vi "Save Load.vi"(6 "error in":errorcluster, 7 "Sub-panel VI names":string[](array[string]), 8 "Temp file path":path=path "D:/control db/control software/Control vi/Temp control/save all temp.txt", 9 "Beamline Section":T1, 10 "Save Load Method":T2, 11 "Sub-panel VI paths array":path[](array[path])) -> (0 "Save Load Error Array Out":errorcluster[](array[cluster]), 2 "Settings Data":cluster{"Name":string, "Variant Data":variant}[](array[cluster]), 3 "Settings Text":string, 4 "enum conversion error array":errorcluster[](array[cluster]))   [LabVIEW 2016, in "Save Load.lvlib"]
doc: "Takes a vi and saves or loads set values depending on which cluster value is chosen"
uses:
  Save Load.lvlib
  save load method.ctl
  beamline selection.ctl
  save or load.ctl
  file or temp.ctl
  all or current.ctl
  main.lvlib
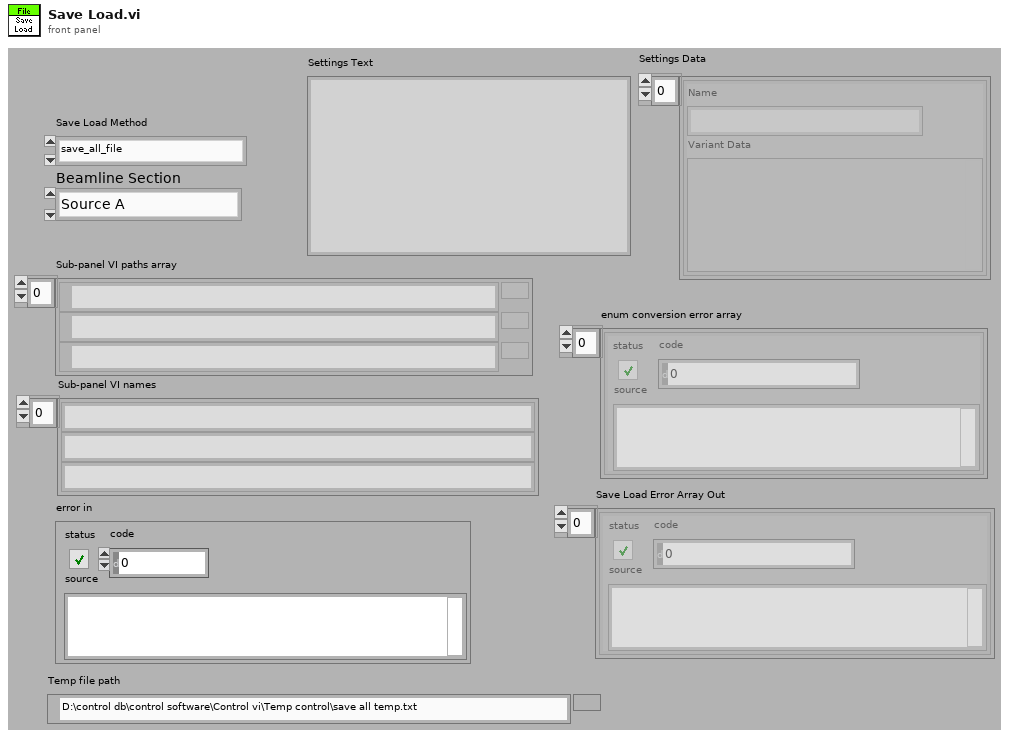
[diagram p1: front panel]
types:
  T1 = typedef "main.lvlib/beamline selection.ctl" = enum16{"Source A", "Source B", "Low Energy End", "High Energy End", "Transmission", "R30", "R45"}
  T2 = typedef "Save Load.lvlib/save load method.ctl" = enum16{"save_all_file", "save_all_temp", "save_curr_file", "save_curr_temp", "load_all_file", "load_all_temp", "load_curr_file", "load_curr_temp"}
  T3 = typedef "Save Load.lvlib/all or current.ctl" = enum16{"current", "all"}
  T4 = typedef "Save Load.lvlib/file or temp.ctl" = enum16{"file", "temp"}
  T5 = typedef "Save Load.lvlib/save or load.ctl" = enum16{"save", "load"}
  T6 = cluster{"format string":string, "format string":string}
  T7 = cluster{"format string":string, "format string":string}[]
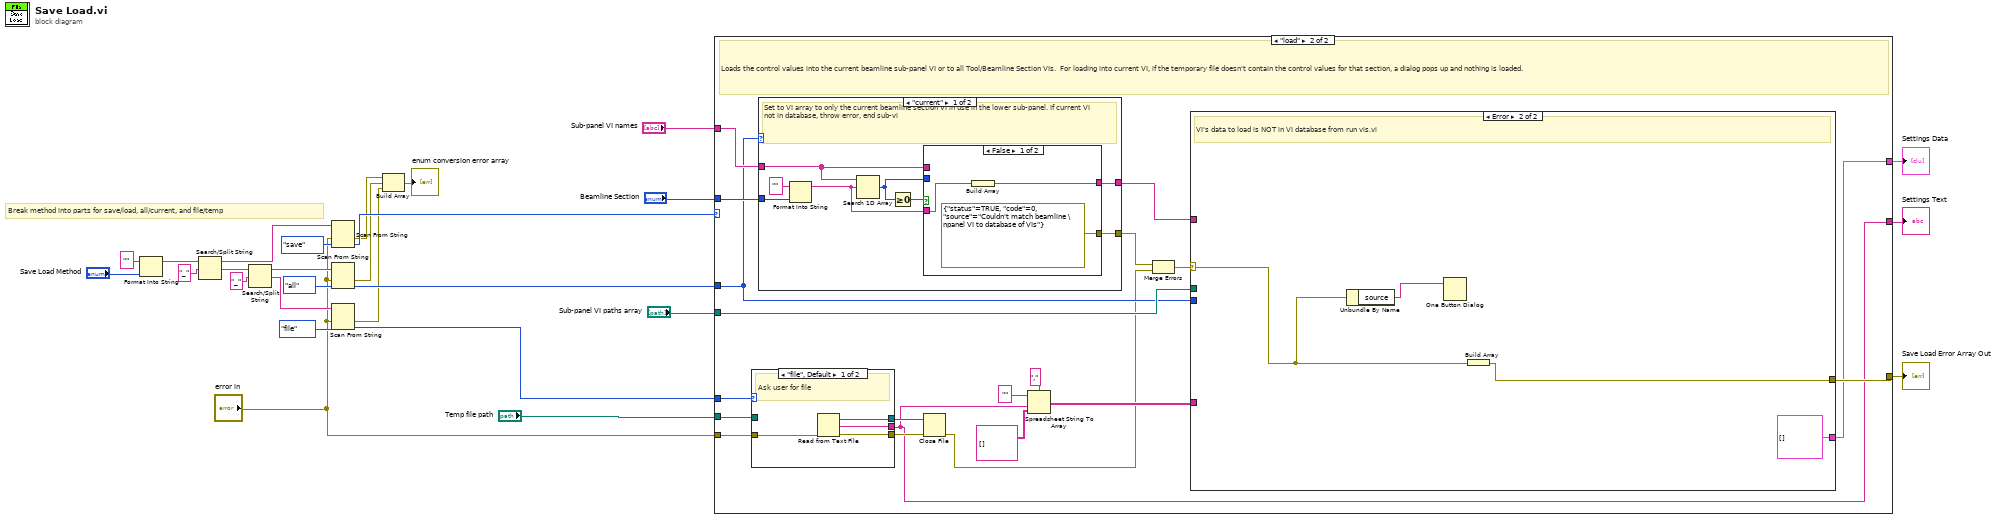
[diagram p0: block diagram]
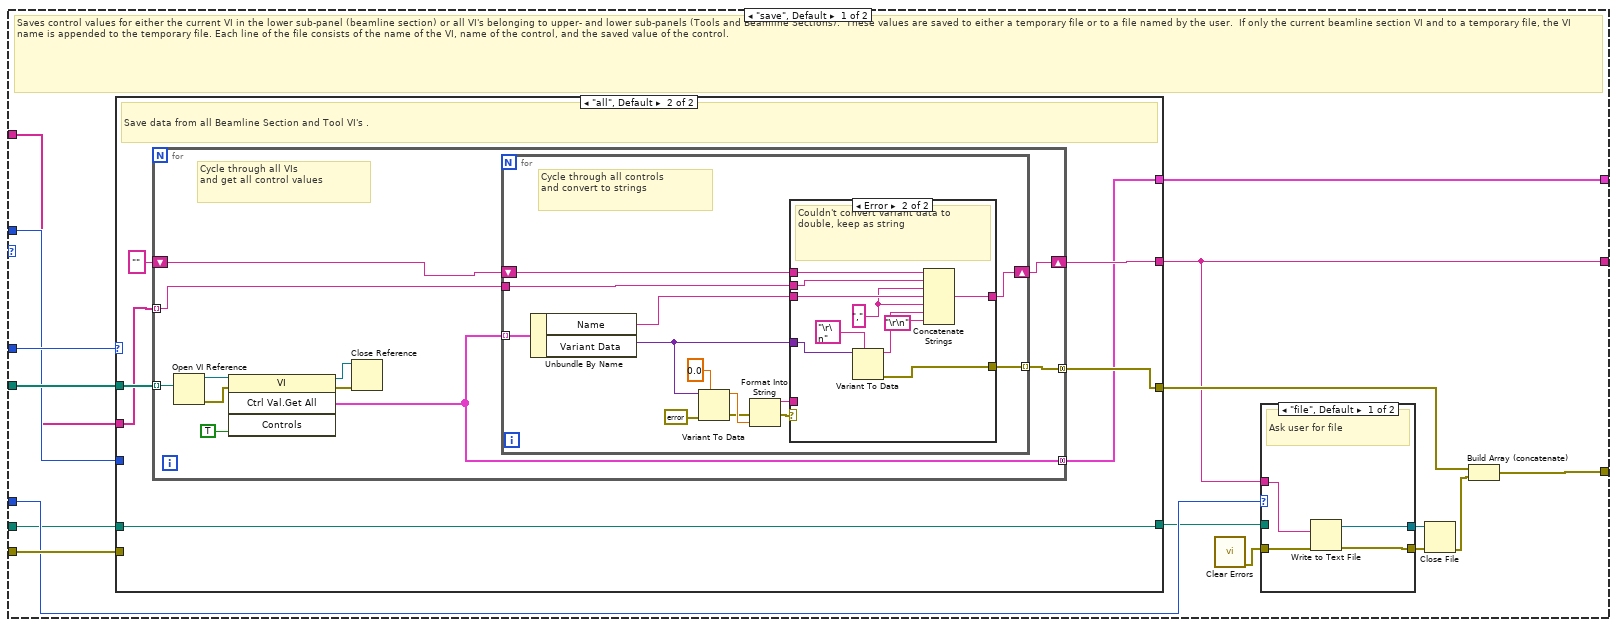
[diagram p2: hidden frame]
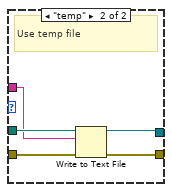
[diagram p3: hidden frame]
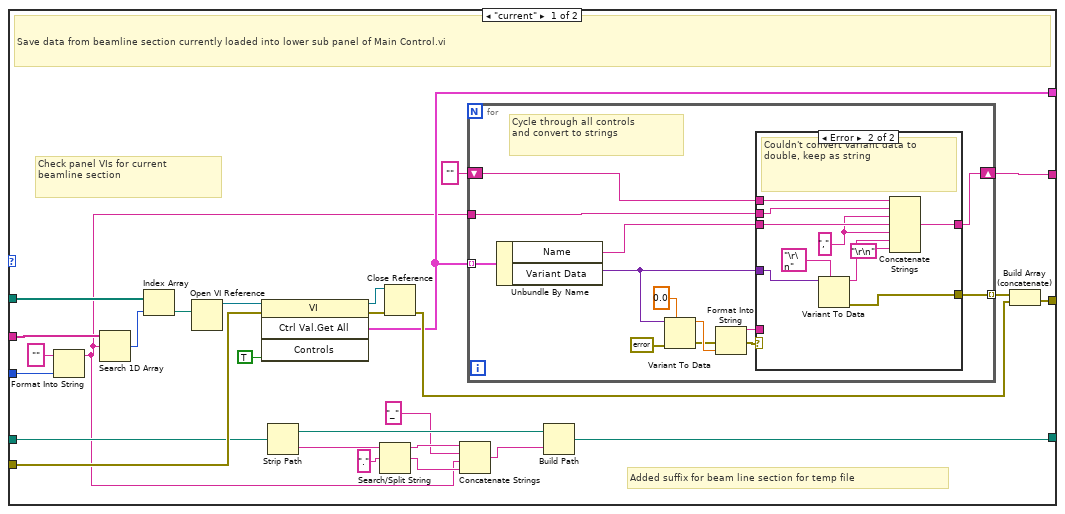
[diagram p4: hidden frame]
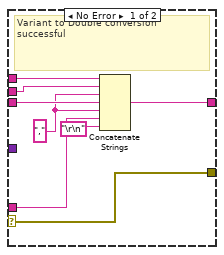
[diagram p5: hidden frame]
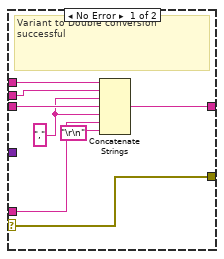
[diagram p6: hidden frame]
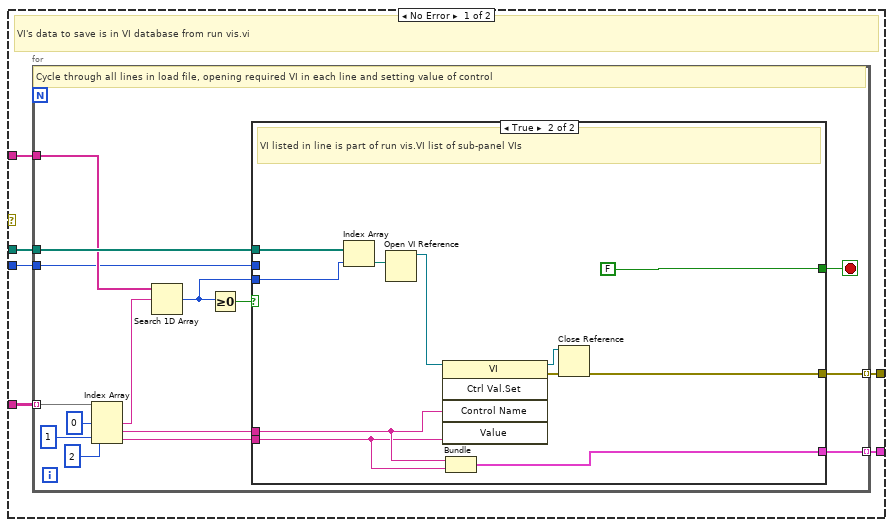
[diagram p7: hidden frame]
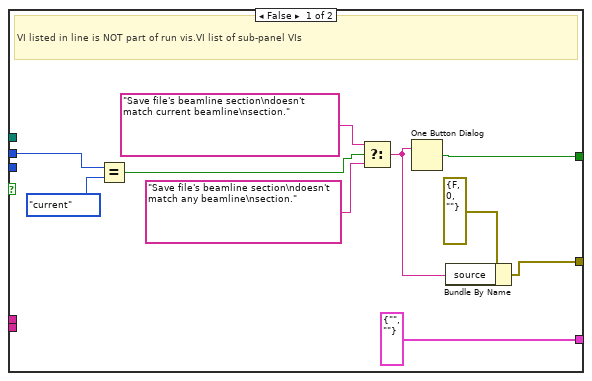
[diagram p8: hidden frame]
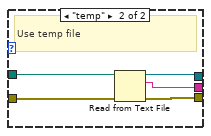
[diagram p9: hidden frame]
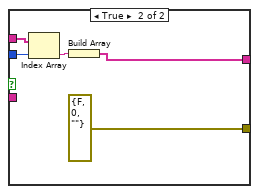
[diagram p10: hidden frame]
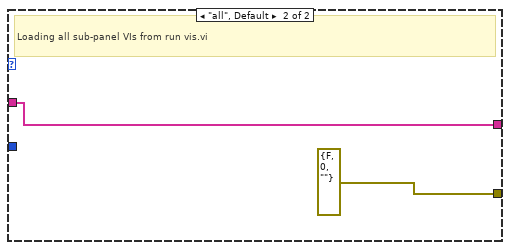
[diagram p11: hidden frame]
diagram:
  # "Break method into parts for save/load, all/current, and file/temp"
  n1 = Format Into String(initial string="", "Save Load Method") -> (resulting string=w24:string)  [unwired: 2 in, 1 out]
  n2 = Search/Split String(string=w24, search string/char (-)="_") -> (substring before match=w19:string, match + rest of string=w25:string)  [unwired: 1 in, 1 out]
  n3 = Search/Split String(string=w25, search string/char (-)="_") -> (substring before match=w18:string, match + rest of string=w17:string)  [unwired: 1 in, 1 out]
  n4 = Scan From String(input string=w19, error in="error in", default 1=save_or_load."save") -> (error out=w13:errorcluster, output 1=w15:T5)  [unwired: 2 in, 2 out]
  n5 = Scan From String(input string=w18, error in="error in", default 1=all_or_current."all") -> (error out=w12:errorcluster, output 1=w14:T3)  [unwired: 2 in, 2 out]
  n6 = Scan From String(input string=w17, error in="error in", default 1=file_or_temp."file") -> (error out=w11:errorcluster, output 1=w9:T4)  [unwired: 2 in, 2 out]
  n7 = Build Array(w13, w12, w11) -> (→"enum conversion error array":errorcluster[])
  n8 = case shown="\"load\"" w15 {
    tunnel: w14 -> [w43 w163]
    tunnel: w9 -> [w30 w179]
    tunnel: "error in" -> [w37 w178]
    tunnel: "Temp file path" -> [w29 w177]
    tunnel: "Sub-panel VI names" -> [w38 w173]
    tunnel: "Sub-panel VI paths array" -> [w40 w168]
    tunnel: "Beamline Section" -> [w39 w174]
    tunnel: [w33 w167] -> w3
    tunnel: [w32 w166] -> w2
    tunnel: [w31 w164] -> w1
    frame "save", Default {
      # "Saves control values for either the current VI in the lower sub-panel (beamline section) or all VI's belonging to upper- and lower sub-panels (Tools and Beamline Sections).  These values are saved to either a temporary file or to a file named by the user.  If only the current beamline section VI and to a temporary file, the VI name is appended to the temporary file. Each line of the file consists of the name of the VI, name of the control, and the saved value of the control."
      n9 = case shown="\"all\", Default" w43 {
        tunnel: w40 -> [w75 w117]
        tunnel: w39 -> [w79 _]
        tunnel: w38 -> [w77 w115]
        tunnel: w37 -> [w63 _]
        tunnel: [w65 w113] -> w34
        tunnel: [w68 w114] -> w32
        tunnel: [w64 w112] -> w31
        tunnel: w29 -> [w62 w111]
        tunnel: [w53 w111] -> w28
        frame "current" {
          # "Check panel VIs for current \nbeamline section"
          # "Added suffix for beam line section for temp file"
          # "Save data from beamline section currently loaded into lower sub panel of Main Control.vi"
          n10 = Format Into String(initial string="", w79) -> (resulting string=w54:string)  [unwired: 2 in, 1 out]
          n11 = Search 1D Array(1D array=w77, element=w54) -> (index of element=w76:i32)  [unwired: 1 in]
          n12 = Index Array(array=w75, index=w76) -> (element=w74:path)
          n13 = Open VI Reference(vi path=w74) -> (vi reference=w73:refnum<vi>)  [unwired: 5 in, 1 out]
          n14 = invoke class="VI" method="Ctrl Val.Get All"(reference=w73, error in=w63, "Controls"=TRUE) -> (reference out=w70:refnum<vi>, error out=w71:errorcluster, "Get All Control Values Variant"=w64:cluster{"Name":string, "Variant Data":variant}[])  [unwired: 1 in, 1 out]
          n15 = Strip Path(path=w62) -> (stripped path=w57:path, name=w61:string)
          n16 = Search/Split String(string=w61, search string/char (-)=".") -> (substring before match=w59:string, match + rest of string=w56:string)  [unwired: 1 in, 1 out]
          n17 = Close Reference(reference=w70, error in (no error)=w71) -> (error out=w66:errorcluster)
          n18 = Concatenate Strings(w59, "_" ("string"), w54, w56) -> (w58:string)
          n19 = for {
            tunnel: w64 -> [w92] mode=indexing
            shift-right: [w86] -> w68
            shift-left: "" -> [w91]
            tunnel: [w82] -> w67 mode=indexing
            tunnel: w54 -> [w81]
            # "Cycle through all controls\nand convert to strings"
            # "Cycle through all the controls on the current beamline section panel"
            n20 = Unbundle By Name(w92) -> ("Name"=w90:string, "Variant Data"=w80:variant)
            n21 = Variant To Data(error in=errorcluster {"status"=FALSE, "code"=0, "source"=""} ("error out"), type=0.0, Variant=w80) -> (data=w88:dbl, error out=w85:errorcluster)
            n22 = Format Into String(error in=w85, w88) -> (resulting string=w87:string, error out=w83:errorcluster)  [unwired: 2 in]
            n23 = case shown="Error" w83 {
              selector: w83 -> [w96 _]
              tunnel: [w99 w105] -> w86
              tunnel: w91 -> [w95 w103]
              tunnel: w90 -> [w98 w106]
              tunnel: w87 -> [w97 _]
              tunnel: w80 -> [_ w109]
              tunnel: [w96 w104] -> w82
              tunnel: w81 -> [w93 w102]
              frame No Error {
                w94 = ","
                # "Variant to Double conversion successful"
                n24 = Concatenate Strings(w95, w93, w94, w98, w94, w97, "\r\n") -> (w99:string)
              }
              frame Error {
                w101 = ","
                # "Couldn't convert variant data to double, keep as string"
                n25 = Variant To Data(type="\r\n", Variant=w109) -> (data=w107:string, error out=w104:errorcluster)  [unwired: 1 in]
                n26 = Concatenate Strings(w103, w102, w101, w106, w101, w107, "\r\n") -> (w105:string)
              }
            }
          }
          n27 = Build Path(base path=w57, name or relative path=w58) -> (appended path=w53:path)
          n28 = Build Array (concatenate)(w67, w66) -> (w65:errorcluster[])
        }
        frame "all", Default {
          # "Save data from all Beamline Section and Tool VI's ."
          n29 = for {
            tunnel: w117 -> [w128] mode=indexing
            shift-right: [w120] -> w114
            shift-left: "" -> [w122]
            tunnel: w115 -> [w121] mode=indexing
            tunnel: [w119] -> w113 mode=concatenating
            tunnel: [w118] -> w112 mode=concatenating
            # "Cycle through all VIs\nand get all control values"
            n30 = Open VI Reference(vi path=w128) -> (vi reference=w124:refnum<vi>, error out=w123:errorcluster)  [unwired: 5 in]
            n31 = invoke class="VI" method="Ctrl Val.Get All"(reference=w124, error in=w123, "Controls"=TRUE) -> (reference out=w125:refnum<vi>, error out=w126:errorcluster, "Get All Control Values Variant"=w118:cluster{"Name":string, "Variant Data":variant}[])  [unwired: 1 in, 1 out]
            n32 = Close Reference(reference=w125, error in (no error)=w126) -> ()  [unwired: 1 out]
            n33 = for {
              tunnel: w118 -> [w141] mode=indexing
              shift-right: [w135] -> w120
              shift-left: w122 -> [w140]
              tunnel: [w131] -> w119 mode=indexing
              tunnel: w121 -> [w130]
              # "Cycle through all controls\nand convert to strings"
              n34 = Unbundle By Name(w141) -> ("Name"=w139:string, "Variant Data"=w129:variant)
              n35 = Variant To Data(error in=errorcluster {"status"=FALSE, "code"=0, "source"=""} ("error out"), type=0.0, Variant=w129) -> (data=w137:dbl, error out=w134:errorcluster)
              n36 = Format Into String(error in=w134, w137) -> (resulting string=w136:string, error out=w132:errorcluster)  [unwired: 2 in]
              n37 = case shown="Error" w132 {
                selector: w132 -> [w145 _]
                tunnel: [w148 w154] -> w135
                tunnel: w140 -> [w144 w152]
                tunnel: w139 -> [w147 w155]
                tunnel: w136 -> [w146 _]
                tunnel: w129 -> [_ w158]
                tunnel: [w145 w153] -> w131
                tunnel: w130 -> [w142 w151]
                frame No Error {
                  w143 = ","
                  # "Variant to Double conversion successful"
                  n38 = Concatenate Strings(w144, w142, w143, w147, w143, w146, "\r\n") -> (w148:string)
                }
                frame Error {
                  w150 = ","
                  # "Couldn't convert variant data to double, keep as string"
                  n39 = Variant To Data(type="\r\n", Variant=w158) -> (data=w156:string, error out=w153:errorcluster)  [unwired: 1 in]
                  n40 = Concatenate Strings(w152, w151, w150, w155, w150, w156, "\r\n") -> (w154:string)
                }
              }
            }
          }
        }
      }
      n41 = call <vilib>:"Clear Errors.vi"() -> ("error out"=w36:errorcluster)  [unwired: 2 in, 5 out]
      n42 = case shown="\"file\", Default" w30 {
        tunnel: [w47 w52] -> w41
        tunnel: w36 -> [w45 w51]
        tunnel: [w46 w50] -> w42
        tunnel: w28 -> [_ w49]
        tunnel: w32 -> [w44 w48]
        frame "file", Default {
          # "Ask user for file"
          n43 = Write to Text File(text=w44, error in=w45) -> (refnum out=w47:refnum<file>, error out=w46:errorcluster)  [unwired: 2 in, 1 out]
        }
        frame "temp" {
          # "Use temp file"
          n44 = Write to Text File(file (use dialog)=w49, text=w48, error in=w51) -> (refnum out=w52:refnum<file>, error out=w50:errorcluster)  [unwired: 1 in, 1 out]
        }
      }
      n45 = Close File(refnum=w41, error in=w42) -> (error out=w35:errorcluster)  [unwired: 1 out]
      n46 = Build Array (concatenate)(w34, w35) -> (w33:errorcluster[])
    }
    frame "load" {
      # "Loads the control values into the current beamline sub-panel VI or to all Tool/Beamline Section VIs.  For loading into current VI, if the temporary file doesn't contain the control values for that section, a dialog pops up and nothing is loaded."
      n47 = case shown="\"file\", Default" w179 {
        tunnel: [w229 w234] -> w175
        tunnel: [w228 w233] -> w166
        tunnel: w178 -> [w226 w232]
        tunnel: [w227 w231] -> w176
        tunnel: w177 -> [_ w230]
        frame "file", Default {
          # "Ask user for file"
          n48 = Read from Text File(error in=w226) -> (refnum out=w229:refnum<file>, text=w228:string, error out=w227:errorcluster)  [unwired: 4 out]
        }
        frame "temp" {
          # "Use temp file"
          n49 = Read from Text File(file (use dialog)=w230, error in=w232) -> (refnum out=w234:refnum<file>, text=w233:string, error out=w231:errorcluster)  [unwired: 3 out]
        }
      }
      n50 = case shown="\"current\"" w163 {
        tunnel: w174 -> [w242 _]
        tunnel: w173 -> [w235 w252]
        tunnel: [w240 w252] -> w169
        tunnel: [w236 errorcluster {"status"=FALSE, "code"=0, "source"=""} ("error constant")] -> w162
        frame "current" {
          # "Set to VI array to only the current beamline section VI in use in the lower sub-panel. If current VI not in database, throw error, end sub-vi"
          n51 = Format Into String(initial string="", w242) -> (resulting string=w237:string)  [unwired: 2 in, 1 out]
          n52 = Search 1D Array(1D array=w235, element=w237) -> (index of element=w239:i32)  [unwired: 1 in]
          n53 = Greater Or Equal To 0?(x=w239) -> (x >= 0?=w238:bool)
          n54 = case shown="False" w238 {
            tunnel: w235 -> [_ w250]
            tunnel: [w245 w248] -> w240
            tunnel: w239 -> [_ w247]
            tunnel: w237 -> [w244 _]
            tunnel: [errorcluster {"status"=TRUE, "code"=0, "source"="Couldn't match beamline \npanel VI to database of VIs"} ("error constant") errorcluster {"status"=FALSE, "code"=0, "source"=""} ("error constant")] -> w236
            frame False {
              n55 = Build Array(w244) -> (w245:string[])
            }
            frame True {
              n56 = Index Array(array=w250, index=w247) -> (element=w249:string)
              n57 = Build Array(w249) -> (w248:string[])
            }
          }
        }
        frame "all", Default {
          # "Loading all sub-panel VIs from run vis.vi"
        }
      }
      n58 = Close File(refnum=w175, error in=w176) -> (error out=w161:errorcluster)  [unwired: 1 out]
      n59 = Spreadsheet String To Array(delimiter (Tab)=",", format string="", spreadsheet string=w166, array type (2D Dbl)=string[][] []) -> (array=w165:string[][])
      n60 = Merge Errors(w162, w161) -> (w160:errorcluster)
      n61 = case shown="Error" w160 {
        selector: w160 -> [_ w224]
        tunnel: w169 -> [w185 _]
        tunnel: w168 -> [w184 _]
        tunnel: [w183 w225] -> w167
        tunnel: w165 -> [w182 _]
        tunnel: [w181 T7 []] -> w164
        tunnel: w163 -> [w180 _]
        frame No Error {
          # "VI's data to save is in VI database from run vis.vi"
          n62 = for {
            tunnel: w182 -> [w200] mode=indexing
            tunnel: w185 -> [w195]
            tunnel: w184 -> [w196]
            tunnel: [w193] -> w183 mode=indexing
            tunnel: [w190] -> w181 mode=indexing
            tunnel: w180 -> [w186]
            stop <- w187 stop-if-true
            # "Cycle through all lines in load file, opening required VI in each line and setting value of control"
            n63 = Index Array(array=w200, index #1=0 ("index"), index #2=1 ("index"), index #3=2 ("index")) -> (element #1=w194:string, element #2=w192:string, element #3=w191:string)
            n64 = Search 1D Array(1D array=w195, element=w194) -> (index of element=w189:i32)  [unwired: 1 in]
            n65 = Greater Or Equal To 0?(x=w189) -> (x >= 0?=w188:bool)
            n66 = case shown="True" w188 {
              tunnel: w196 -> [_ w220]
              tunnel: [w201 w216] -> w193
              tunnel: w192 -> [_ w215]
              tunnel: w191 -> [_ w214]
              tunnel: [T6 {"format string"="", "format string"=""} w213] -> w190
              tunnel: w189 -> [_ w212]
              tunnel: [w209 FALSE] -> w187
              tunnel: w186 -> [w206 _]
              frame False {
                # "VI listed in line is NOT part of run vis.VI list of sub-panel VIs"
                n67 = Equal?(x=w206, y=all_or_current."current") -> (x = y?=w205:bool)
                n68 = Select(t="Save file's beamline section\ndoesn't match current beamline\nsection.", s=w205, f="Save file's beamline section\ndoesn't match any beamline\nsection.") -> (s? t:f=w202:string)
                n69 = One Button Dialog(message=w202) -> (true=w209:bool)  [unwired: 1 in]
                n70 = Bundle By Name(cluster=errorcluster {"status"=FALSE, "code"=0, "source"=""} ("error out"), "source"=w202) -> (w201:errorcluster)
              }
              frame True {
                # "VI listed in line is part of run vis.VI list of sub-panel VIs"
                n71 = Index Array(array=w220, index=w212) -> (element=w221:path)
                n72 = Open VI Reference(vi path=w221) -> (vi reference=w219:refnum<vi>)  [unwired: 5 in, 1 out]
                n73 = invoke class="VI" method="Ctrl Val.Set"(reference=w219, "Control Name"=w215, "Value"=w214) -> (reference out=w217:refnum<vi>, error out=w218:errorcluster)  [unwired: 2 in, 3 out]
                n74 = Bundle("format string"=w215, "format string"=w214) -> (w213:T6)  [unwired: 1 in]
                n75 = Close Reference(reference=w217, error in (no error)=w218) -> (error out=w216:errorcluster)
              }
            }
          }
        }
        frame Error {
          # "VI's data to load is NOT in VI database from run vis.vi"
          n76 = Unbundle By Name(w224) -> ("source"=w223:string)
          n77 = One Button Dialog(message=w223) -> ()  [unwired: 1 in, 1 out]
          n78 = Build Array(w224) -> (w225:errorcluster[])
        }
      }
    }
  }
  "Save Load Error Array Out" <- w3
  "Settings Text" <- w2
  "Settings Data" <- w1
